vi "Write Protocols.vi"(8 "error in (no error)":errorcluster, 10 "Protocols":string[](array[string]), 11 "WebSocket in":refnum<class "WebSocket.lvclass">) -> (0 "error out":errorcluster, 3 "WebSocket out":refnum<class "WebSocket.lvclass">)   [LabVIEW 2013, in "WebSockets.lvlib" / "WebSocket.lvclass"]
uses:
  WebSocket.lvclass
  WebSocket.lvclass/WebSocket.ctl
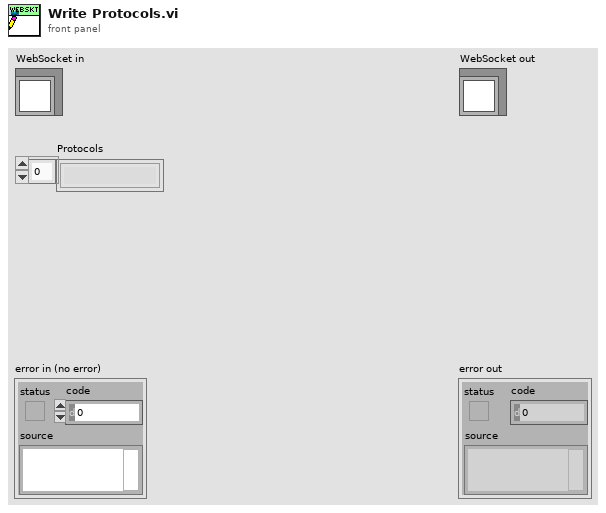
[diagram p1: front panel]
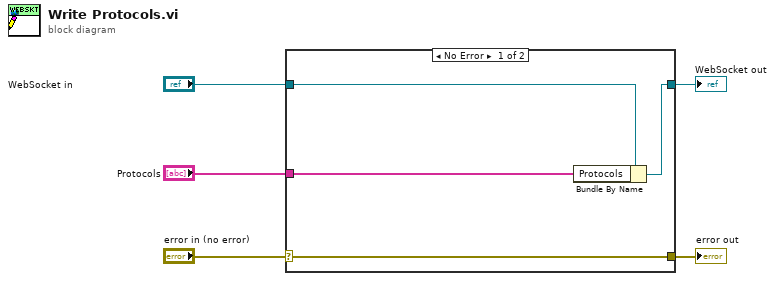
[diagram p0: block diagram]
diagram:
  n1 = case shown="No Error" "error in (no error)" {
    selector: "error in (no error)" -> [w9 w10]
    tunnel: [w9 w10] -> w4
    tunnel: [w7 w11] -> w2
    tunnel: "WebSocket in" -> [w8 w11]
    tunnel: "Protocols" -> [w6 _]
    frame No Error {
      n2 = Bundle By Name(cluster=w8, "Protocols"=w6) -> (w7:refnum<class "WebSocket.lvclass">)
    }
    frame Error {
    }
  }
  "error out" <- w4
  "WebSocket out" <- w2
